vi "EXAMPLE_TAGDBDEMO.vi"() -> ()   [LabVIEW 2014]
uses:
  TagDB/_Support/Access/_setAnything.vi
  TagDB/_Support/Properties/tagDB dbChanged.vi
  TagDB/_Support/Access/_variant.vi
  TagDB/_Support/Error/_[error50002]Invalid DataType.vi
  TagDB/_Support/Private/_Cast TagDB Ref to DVR.vi
  TagDB/_Support/Error/_[error50000]Invalid DB REF.vi
  TagDB/_XNode/tagDB_setValue.xnode/tagDB_setValue.xnode
  TagDB/tagDB_Def.ctl
  TagDB/_XNode/tagDB_value.xnode/tagDB_value.xnode
  TagDB/TagDB(dev).lvlib
panel:
  out "Not Predef Tag":string
  out "value 2":variant
  out "DataItemFlag":i64
  out "DataChangeFlag":i64
  in  "value":string="test send message"
  out "String":string
  in  "stop":bool
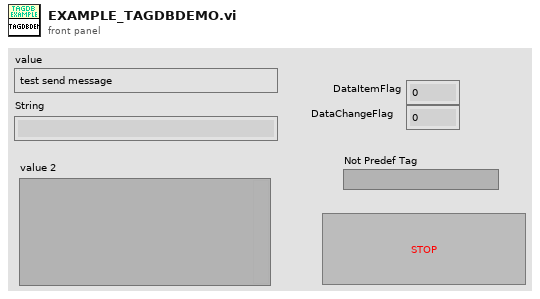
[diagram p1: front panel]
types:
  T1 = cluster{"number":i32, "boolean":bool, "abcdef":cluster{"number":i32, "boolean":bool}}
  T2 = typedef "TagDB(dev).lvlib/tagDB_Def.ctl" = refnum<k1>
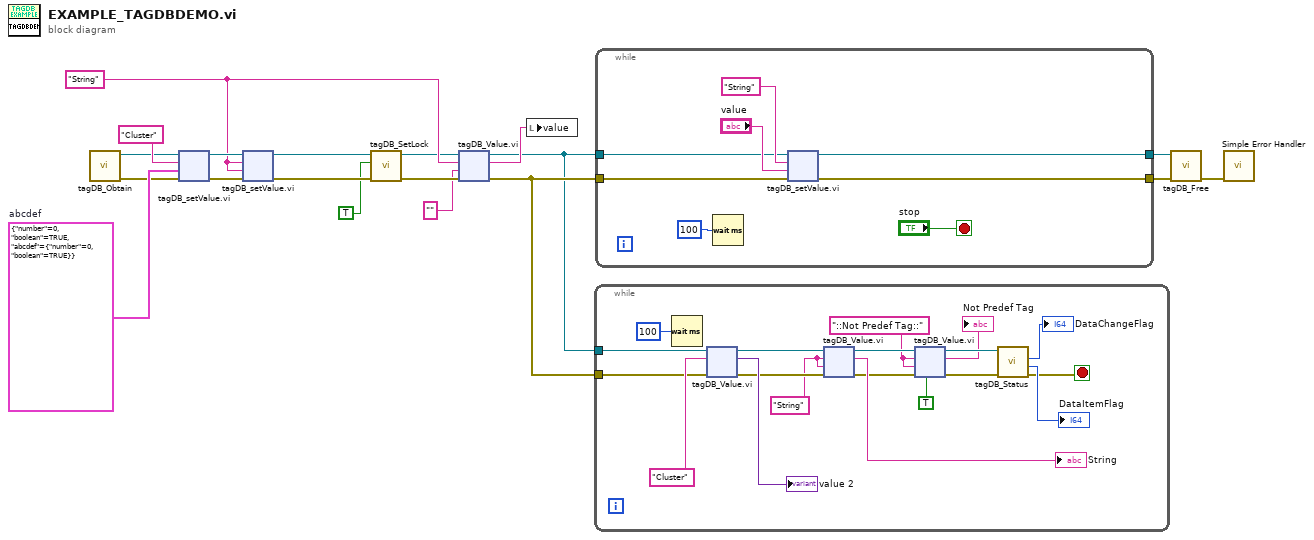
[diagram p0: block diagram]
diagram:
  w11 = T1 {"number"=0, "boolean"=TRUE, "abcdef"={"number"=0, "boolean"=TRUE}}  # abcdef
  w8 = "String" ("String")
  n1 = call "tagDB_Obtain.vi"() -> ("error out"=w10:errorcluster, "DB"=w2:T2)  [unwired: 5 in, 1 out]
  n2 = xnode "tagDB_setValue.vi"("DB Ref"=w2, "name"="Cluster", "value"=w11, "Error In"=w10) -> ("DB Ref(dup)"=w14:T2, "Error Out"=w13:errorcluster)  [unwired: 1 out]
  n3 = xnode "tagDB_setValue.vi"("DB Ref"=w14, "name"=w8, "value"=w8, "Error In"=w13) -> ("DB Ref(dup)"=w15:T2, "Error Out"=w6:errorcluster)  [unwired: 1 out]
  n4 = call "tagDB_SetLock.vi"("error in (no error)"=w6, "Lock?"=TRUE, "DB Ref"=w15) -> ("error out"=w5:errorcluster, "DB Ref(dup)"=w7:T2)  [unwired: 7 in]
  n5 = xnode "tagDB_Value.vi"("error in (no error)"=w5, "DB Ref"=w7, "Type"="", "name"=w8) -> ("error out"=w17:errorcluster, "DB Ref(dup)"=w1:T2, "value"=w16:string)  [unwired: 1 in]
  n6 = local write "value"(w16) -> ()
  n7 = while {
    tunnel: w1 -> [w31]
    tunnel: w17 -> [w29]
    stop <- w32 stop-if-true
    w20 = "::Not Predef Tag::" ("name")
    w27 = "String" ("name")
    n8 = Wait (ms)(milliseconds to wait=u32 100) -> ()  [unwired: 1 out]
    n9 = xnode "tagDB_Value.vi"("error in (no error)"=w29, "DB Ref"=w31, "name"="Cluster") -> ("error out"=w28:errorcluster, "DB Ref(dup)"=w30:T2, "value"=→"value 2":variant)  [unwired: 2 in]
    n10 = xnode "tagDB_Value.vi"("error in (no error)"=w28, "DB Ref"=w30, "Type"=w27, "name"=w27) -> ("error out"=w25:errorcluster, "DB Ref(dup)"=w26:T2, "value"=→"String":string)  [unwired: 1 in]
    n11 = xnode "tagDB_Value.vi"("error in (no error)"=w25, "DB Ref"=w26, "Type"=w20, "Add wih NonExist?"=TRUE, "name"=w20) -> ("error out"=w24:errorcluster, "DB Ref(dup)"=w23:T2, "value"=→"Not Predef Tag":string)
    n12 = call "tagDB_Status.vi"("error in (no error)"=w24, "DB Ref"=w23) -> ("error out"=w32:errorcluster, "#Item Change"=→"DataItemFlag":i64, "#Data Change"=→"DataChangeFlag":i64)  [unwired: 4 in, 3 out]
  }
  n13 = while {
    tunnel: w1 -> [w176]
    tunnel: w17 -> [w177]
    tunnel: [w175] -> w9
    tunnel: [w178] -> w18
    stop <- "stop" stop-if-true
    n14 = Wait (ms)(milliseconds to wait=u32 100) -> ()  [unwired: 1 out]
    n15 = xnode "tagDB_setValue.vi"("DB Ref"=w176, "name"="String", "value"="value", "Error In"=w177) -> ("DB Ref(dup)"=w178:T2, "Error Out"=w175:errorcluster)  [unwired: 1 out]
  }
  n16 = call "tagDB_Free.vi"("error in (no error)"=w9, "DB Ref"=w18) -> ("error out"=w19:errorcluster)  [unwired: 9 in]
  n17 = call <vilib>:"Simple Error Handler.vi"("error in (no error)"=w19) -> ()  [unwired: 4 in, 5 out]
